vi "PostUserData.vi"() -> ()   [LabVIEW 2025]
doc: "Sends a POST API request with user data including name, ID, email, password, and role. The response from the server is captured and stored in a response body string."
uses:
  <vilib>/httpClient/POSTBuffer.vi
  <vilib>/httpClient/LabVIEWHTTPClient.lvlib
panel:
  out "response body":string
  in  "User":T1
  # "Made post api request by sending user data and getting response to response body string"
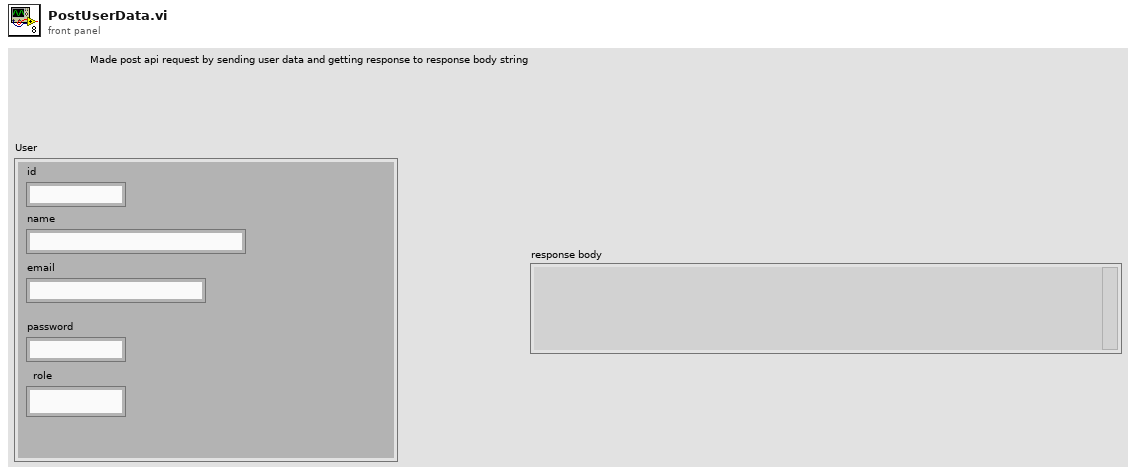
[diagram p1: front panel]
types:
  T1 = cluster{"id":string, "name":string, "email":string, "password":string, "role":string}
  T2 = typedef "LabVIEWHTTPClient.lvlib/ClientHandle.ctl" = refnum<k1>
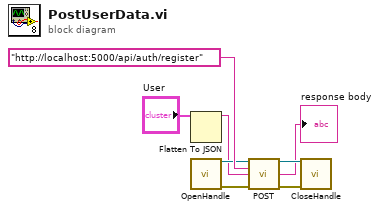
[diagram p0: block diagram]
diagram:
  n1 = Flatten To JSON(anything="User") -> (JSON string=w3:string)  [unwired: 2 in, 1 out]
  n2 = call <vilib>:"OpenHandle.vi"() -> ("client handle out"=w6:T2, "error out"=w7:errorcluster)  [unwired: 14 in]
  n3 = call-poly <vilib>:"POST.vi"("client handle"=w6, "url"="http://localhost:5000/api/auth/register", "buffer"=w3, "error in (no error)"=w7) -> ("client handle out"=w5:T2, "body"=→"response body":string, "error out"=w4:errorcluster)  [unwired: 8 in, 1 out]
  n4 = call <vilib>:"CloseHandle.vi"("client handle"=w5, "error in (no error)"=w4) -> ()  [unwired: 13 in, 1 out]
